vi "set_timeouts.vi"(5 "read_timeout (ms); def=1000":i32=1000, 7 "write_timeout (ms); def=1000":i32=1000, 11 "error in (no error)":errorcluster) -> (15 "error out":errorcluster)   [LabVIEW 2012]
doc: "Sets both USB read and write timeouts (in milliseconds). \n\nImplementss the USB Communication API function \"fnPerformaxComSetTimeouts\". \n\nThe command is an enumerated constant containing all the commands supported by the LabVIEW USB Communication driver. All commands covered here can be mapped to the commands outlined in the ASCII Language Specification of the USB Communication API documenation.\n\nIf the \"command (raw)\" field is not empty, this VI assumes the user has chosen to send a raw command as outlined in the ASCII Language Specification of the USB Communication API documentation. The \"command\" input field will be ignored.\n\nProduced By:\n\nChristopher Lemieux\nKod Integrations, LLC\n4835 Marianne Drive\nMount Airy, MD 21771\nhttp://www.kodintegrations.com\nemail: clemieux@kodintegrations.com\nphone: (240) 687-1288"
uses:
  support/controls/errors_actions.ctl
  PerformaxCom.dll
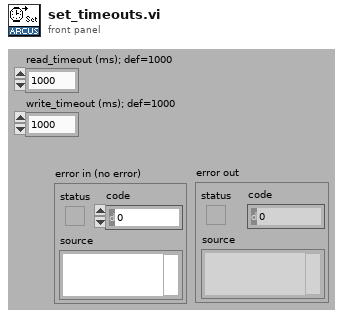
[diagram p1: front panel]
types:
  T1 = typedef "errors_actions.ctl" = enum16{"clearBuff", "closeRef", "noDeviceInfo", "noDevices", "openRef", "sendReceive", "setTimeouts", "unknown"}
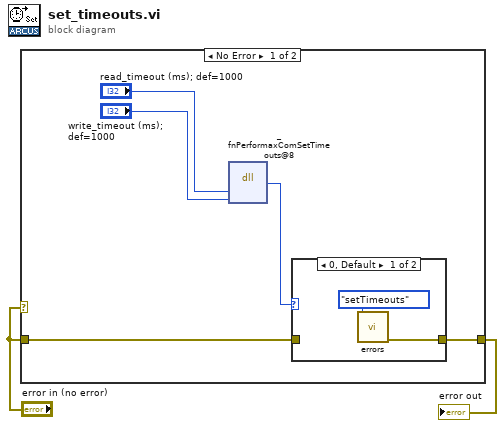
[diagram p0: block diagram]
diagram:
  n1 = case shown="No Error" "error in (no error)" {
    tunnel: "error in (no error)" -> [w6 w11]
    tunnel: [w5 w11] -> w1
    frame No Error {
      n2 = dll-call lib="PerformaxCom.dll" fn="_fnPerformaxComSetTimeouts@8"("readTimeout"="read_timeout (ms); def=1000", "writeTimeout"="write_timeout (ms); def=1000") -> (w7:i32)  [unwired: 5 in, 2 out]
      n3 = case shown="0, Default" w7 {
        tunnel: [w8 w10] -> w5
        tunnel: w6 -> [_ w10]
        frame 0, Default {
          n4 = call "errors.vi"("errors"=errors_actions."setTimeouts") -> ("error out"=w8:errorcluster)  [unwired: 14 in]
        }
        frame 1 {
        }
      }
    }
    frame Error {
    }
  }
  "error out" <- w1
